vi "mj_getTermID.vi"(9 "Data type":T1=enum."Data Object") -> (3 "terminal ID":string)   [LabVIEW 2017]
uses:
  <vilib>/Platform/storage/lvStorage.llb/_dataTypeEnumForTerminals.ctl
panel:
  in  "Name":string[](array[string])=["storage refnum", "storage refnum", "storage refnum (file)", "storage refnum (channel)", "error in (no error)", "error out", "file path", "storage location", "storage format", "function (open:0)", "append / replace (append data values)", "index", "count", "comparison", "Signal", "storage refnum (channel group)", "Cluster", "DBL", "SGL", "I32", "I16", "U8", "TIME", "STRING", "ENUM", "waveform", "DDT", "DAQmx Task"]
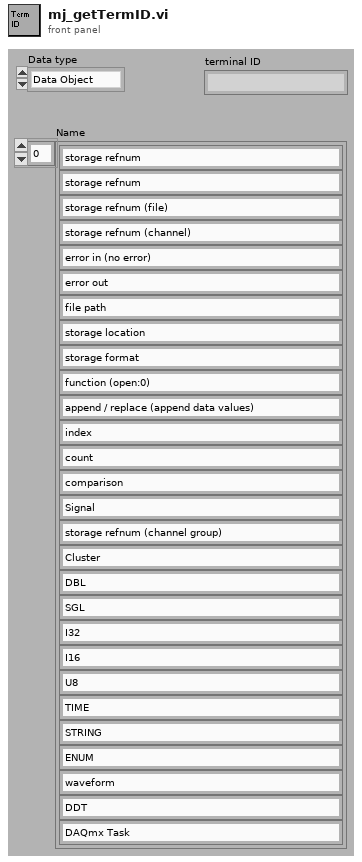
[diagram p1: front panel]
types:
  T1 = typedef "_dataTypeEnumForTerminals.ctl" = enum16{"Data Storage", "Data Object", "Root", "Channel", "Error in", "Error out", "Storage Location (path)", "Storage Location (string)", "Storage Format", "Overwrite options (enum)", "Append / Replace (enum)", "index", "count", "Comparison (enum)", "Signal", "Channelgroup", "Cluster", "DBL", "SGL", "I32", "I16", "U8", "TIME", "STRING", "ENUM", "waveform", "DDT", "DAQmx Channel"}
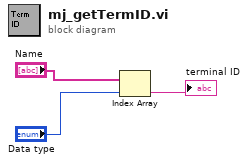
[diagram p0: block diagram]
diagram:
  n1 = Index Array(array="Name", index="Data type") -> (element=→"terminal ID":string)
